vi "disconnect.vi"(8 "error in (no error)":errorcluster, 11 "TCPClient in":refnum<class "TCPClient.lvclass">) -> (0 "error out":errorcluster, 3 "TCPClient out":refnum<class "TCPClient.lvclass">, 4 "error diconnect":errorcluster)   [LabVIEW 2016, in "tcp.lvlib" / "TCPClient.lvclass"]
uses:
  TCPClient.lvclass
  TCPClient.lvclass/TCPClient.ctl
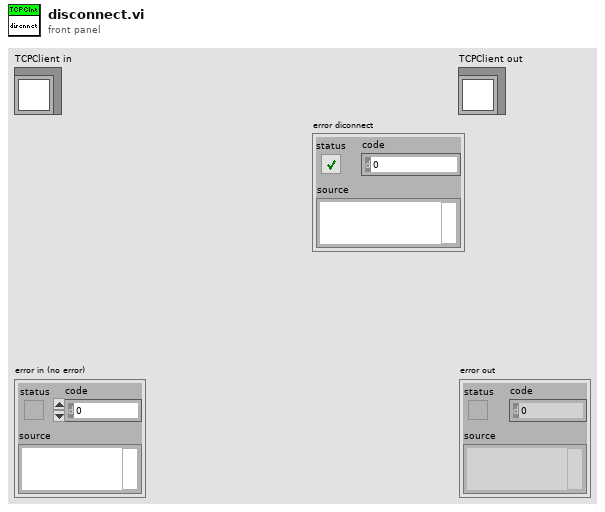
[diagram p1: front panel]
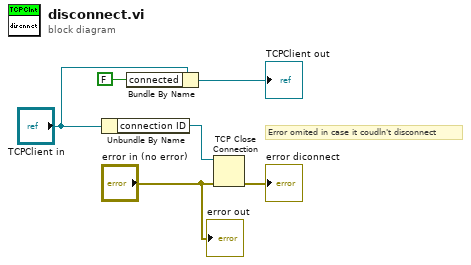
[diagram p0: block diagram]
diagram:
  # "Error omited in case it coudln't disconnect"
  n1 = Unbundle By Name("TCPClient in") -> ("connection ID"=w6:refnum<k5>)
  n2 = Bundle By Name(cluster="TCPClient in", "connected"=FALSE) -> (→"TCPClient out":refnum<class "TCPClient.lvclass">)
  n3 = TCP Close Connection(connection ID=w6, error in (no error)="error in (no error)") -> (error out=→"error diconnect":errorcluster)  [unwired: 2 out]
  "error out" <- "error in (no error)"
